vi "PATH STRIP.vi"(11 "path":path) -> (3 "appended path":path)   [LabVIEW 2018]
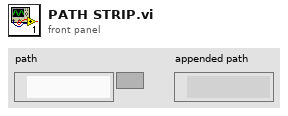
[diagram p1: front panel]
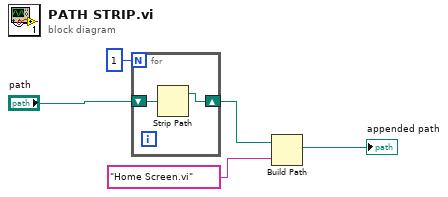
[diagram p0: block diagram]
diagram:
  n1 = for {
    N: 1 -> [_]
    shift-right: [w6] -> w2
    shift-left: "path" -> [w7]
    n2 = Strip Path(path=w7) -> (stripped path=w6:path)  [unwired: 1 out]
  }
  n3 = Build Path(base path=w2, name or relative path="Home Screen.vi") -> (appended path=→"appended path":path)
